vi "custom_2_stimulus_generator.vi"(1 "input cluster":T1) -> (0 "output cluster":cluster{i32, i32, "Elapsed Time":i32})   [LabVIEW 2015]
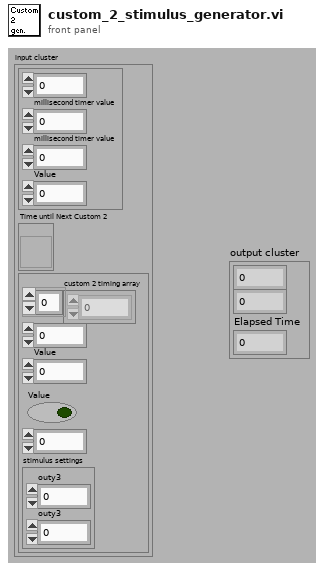
[diagram p1: front panel]
types:
  T1 = cluster{cluster{u32, "millisecond timer value":u32, "millisecond timer value":u32, "Value":u32}, "Time until Next Custom 2":refnum<vi>, cluster{"custom 2 timing array":dbl[], i32, "Value":i32, "Value":bool, i32, "stimulus settings":cluster{"outy3":sgl, "outy3":i32}}}
  T2 = cluster{u32, "millisecond timer value":u32, "millisecond timer value":u32, "Value":u32}
  T3 = cluster{"custom 2 timing array":dbl[], i32, "Value":i32, "Value":bool, i32, "stimulus settings":cluster{"outy3":sgl, "outy3":i32}}
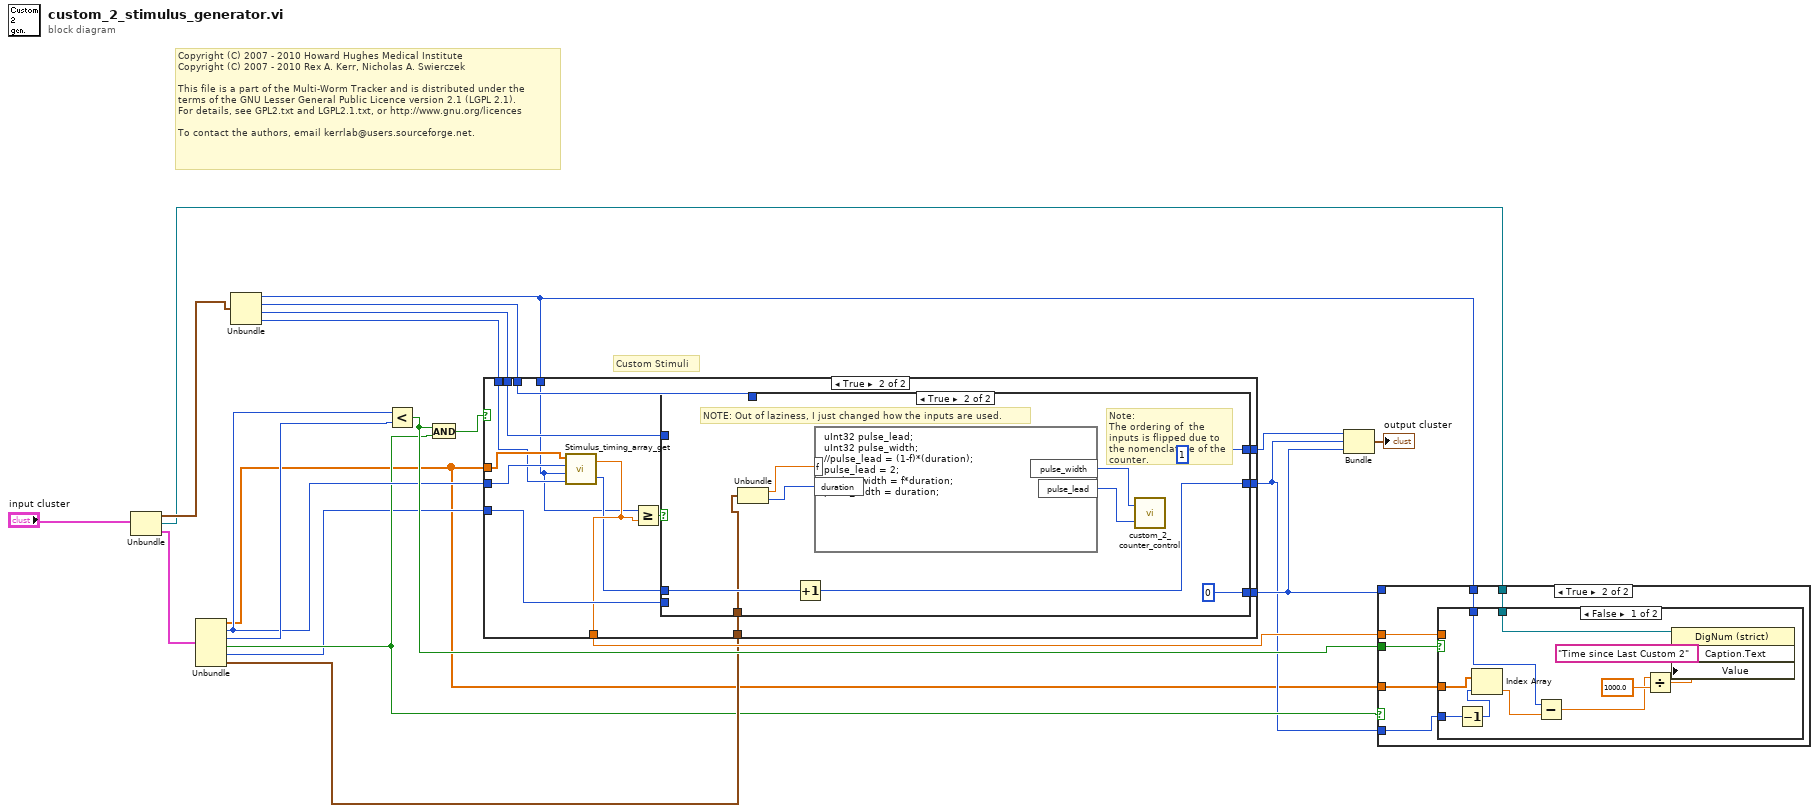
[diagram p0: block diagram]
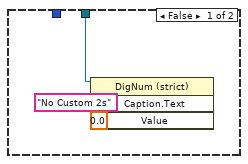
[diagram p2: hidden frame]
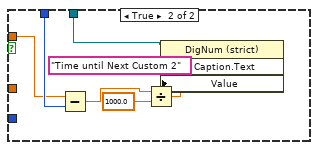
[diagram p3: hidden frame]
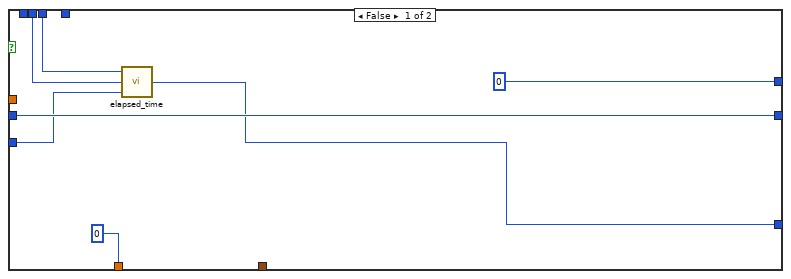
[diagram p4: hidden frame]
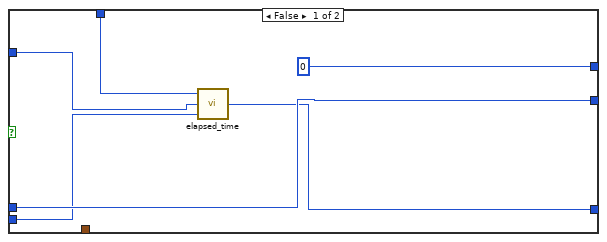
[diagram p5: hidden frame]
diagram:
  # "Copyright (C) 2007 - 2010 Howard Hughes Medical Institute\nCopyright (C) 2007 - 2010 Rex A. Kerr, Nicholas A. Swierczek\n \nThis file is a part of the Multi-Worm Tracker and is distributed under the\nterms of the GNU Lesser General Public Licence version 2.1 (LGPL 2.1).\nFor details, see GPL2.txt and LGPL2.1.txt, or http://www.gnu.org/licences\n \nTo contact the authors, email kerrlab@users.sourceforge.net."
  # "Custom Stimuli"
  n1 = Unbundle("input cluster") -> (w18:T2, "Time until Next Custom 2"=w15:refnum<vi>, w17:T3)
  n2 = Unbundle(w17) -> ("custom 2 timing array"=w1:dbl[], w13:i32, "Value"=w14:i32, "Value"=w12:bool, w11:i32, "stimulus settings"=w16:cluster{"outy3":sgl, "outy3":i32})
  n3 = Unbundle(w18) -> (w3:u32, "millisecond timer value"=w5:u32, "millisecond timer value"=w6:u32, "Value"=w4:u32)
  n4 = Less?(x=w13, y=w14) -> (x < y?=w20:bool)
  n5 = And(x=w20, y=w12) -> (x .and. y?=w21:bool)
  n6 = case shown="True" w21 {
    tunnel: w1 -> [_ w32]
    tunnel: w13 -> [w28 w31]
    tunnel: [w28 w40] -> w2
    tunnel: w11 -> [w23 w36]
    tunnel: [w22 w41] -> w9
    tunnel: w5 -> [w25 w39]
    tunnel: w6 -> [w24 w38]
    tunnel: [0 w37] -> w10
    tunnel: [0 w34] -> w19
    tunnel: w16 -> [_ w35]
    tunnel: w3 -> [_ w29]
    tunnel: w4 -> [_ w30]
    frame False {
      n7 = call "elapsed_time.vi"("Time since last update"=w23, "Initial Time"=w24, "Current Time"=w25) -> ("Elapsed Time"=w22:i32)
    }
    frame True {
      n8 = call "Stimulus_timing_array_get.vi"("minimum time between events"=w30, "experiment time"=w29, "array index"=w31, "timing array"=w32) -> ("index"=w33:i32, "time"=w34:dbl)
      n9 = Greater Or Equal?(x=w29, y=w34) -> (x >= y?=w42:bool)
      n10 = case shown="True" w42 {
        tunnel: [w46 0] -> w41
        tunnel: w33 -> [w48 w56]
        tunnel: [w48 w55] -> w40
        tunnel: w36 -> [w45 _]
        tunnel: w39 -> [w43 _]
        tunnel: w38 -> [w44 _]
        tunnel: [0 1] -> w37
        tunnel: w35 -> [_ w53]
        frame False {
          n11 = call "elapsed_time.vi"("Time since last update"=w45, "Initial Time"=w44, "Current Time"=w43) -> ("Elapsed Time"=w46:i32)
        }
        frame True {
          # "Note:\nThe ordering of  the\ninputs is flipped due to \nthe nomenclature of the counter."
          # "NOTE: Out of laziness, I just changed how the inputs are used."
          n12 = Unbundle(w53) -> ("outy3"=w52:sgl, "outy3"=w51:i32)
          n13 = Increment(x=w56) -> (x+1=w55:i32)
          n14 = formula code="uInt32 pulse_lead;\nuInt32 pulse_width;\n//pulse_lead = (1-f)*(duration);\npulse_lead = 2;\n//pulse_width = f*duration;\npulse_width = duration;"("f"=w52, "duration"=w51) -> ("pulse_lead"=w49:u32, "pulse_width"=w50:u32)
          n15 = call "custom_2_counter_control.vi"("Signal-high duration"=w49, "Signal-high lead-up"=w50) -> ()
        }
      }
    }
  }
  n16 = Bundle(w10, "index"=w2, "Elapsed Time"=w9) -> (→"output cluster":cluster{i32, "index":i32, "Elapsed Time":i32})  [unwired: 1 in]
  n17 = case shown="True" w12 {
    tunnel: w20 -> [_ w66]
    tunnel: w19 -> [_ w65]
    tunnel: w9 -> [_ _]
    tunnel: w15 -> [w58 w64]
    tunnel: w3 -> [_ w63]
    tunnel: w2 -> [_ w62]
    tunnel: w1 -> [_ w61]
    frame False {
      n18 = property on="Property Node" class="DigNum (strict)"(reference=w58, "Caption.Text"="No Custom 2s" ("Label.Text"), "Value"=0.0 ("Time until Next Puff")) -> ()  [unwired: 1 in, 2 out]
    }
    frame True {
      n19 = case shown="False" w66 {
        tunnel: w65 -> [_ w81]
        tunnel: w63 -> [w68 w82]
        tunnel: w64 -> [w73 w77]
        tunnel: w62 -> [w72 _]
        tunnel: w61 -> [w70 _]
        frame False {
          n20 = Decrement(x=w72) -> (x-1=w71:i32)
          n21 = Index Array(array=w70, index=w71) -> (element=w69:dbl)
          n22 = Subtract(x=w68, y=w69) -> (x-y=w67:dbl)
          n23 = Divide(x=w67, y=1000.0) -> (x/y=w74:dbl)
          n24 = property on="Property Node" class="DigNum (strict)"(reference=w73, "Caption.Text"="Time since Last Custom 2" ("Label.Text"), "Value"=w74) -> ()  [unwired: 1 in, 2 out]
        }
        frame True {
          n25 = Subtract(x=w81, y=w82) -> (x-y=w79:dbl)
          n26 = Divide(x=w79, y=1000.0) -> (x/y=w78:dbl)
          n27 = property on="Property Node" class="DigNum (strict)"(reference=w77, "Caption.Text"="Time until Next Custom 2" ("Label.Text"), "Value"=w78) -> ()  [unwired: 1 in, 2 out]
        }
      }
    }
  }
